vi "WheelSpinnerActions.vi"() -> ()   [LabVIEW 2019]
panel:
  in  "Cluster":T1
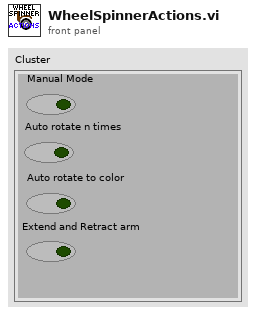
[diagram p1: front panel]
types:
  T1 = cluster{"Manual Mode":bool, "Auto rotate n times":bool, "Auto rotate to color":bool, "Extend and Retract arm":bool}
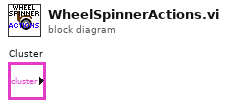
[diagram p0: block diagram]
diagram:
